vi "Write Nested Libraries.vi"(8 "error in (no error)":errorcluster, 10 "Nested Libraries":T1[](array[typedef]), 11 "TAF Proj Document Type:FrontPanelGUI in":refnum<class "FrontPanelGUI.lvclass">) -> (0 "error out":errorcluster, 3 "TAF Proj Document Type:FrontPanelGUI out":refnum<class "FrontPanelGUI.lvclass">)   [LabVIEW 2021]
uses:
  <vilib>/Wovalab/AntiDoc/Document Type/Add-ons/LabVIEW YAF Project/FrontPanelGUI/FrontPanelGUI.lvclass
  C:/Program Files (x86)/National Instruments/LabVIEW 2021/vi.lib/Wovalab/AntiDoc/Bloc/Bloc.lvclass
  C:/Program Files (x86)/National Instruments/LabVIEW 2021/vi.lib/Wovalab/AntiDoc/Document Type/Add-ons/LabVIEW YAF Project/FrontPanelGUI/FrontPanelGUI.lvclass
  <vilib>/Wovalab/AntiDoc/Document Type/Add-ons/LabVIEW YAF Project/FrontPanelGUI/Nested Lib Info--cluster.ctl
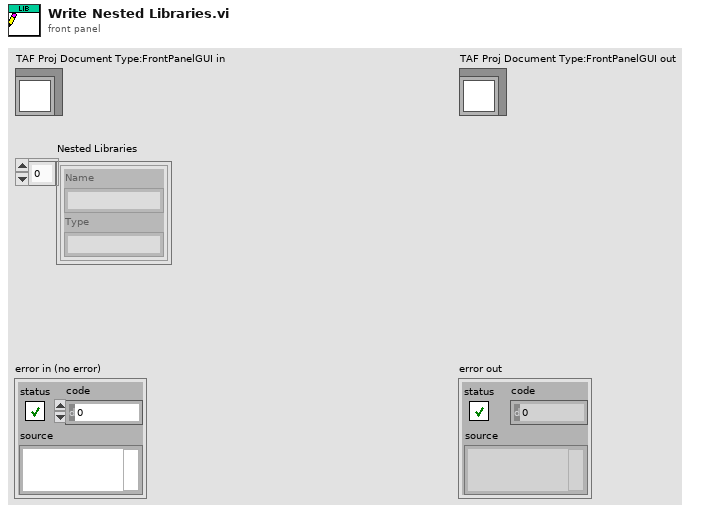
[diagram p1: front panel]
types:
  T1 = typedef "TAF Proj Document Type.lvlib/FrontPanelGUI.lvclass/Nested Lib Info--cluster.ctl" = cluster{"Name":string, "Type":string}
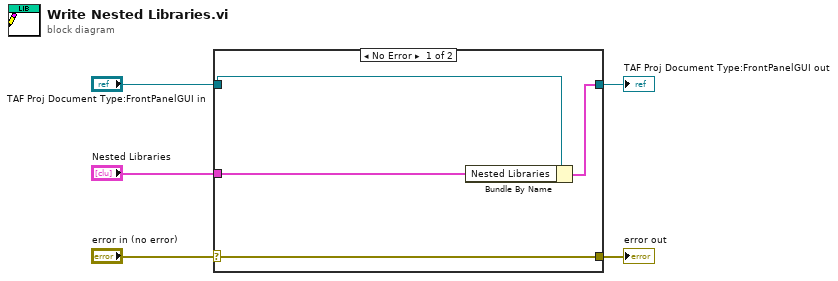
[diagram p0: block diagram]
diagram:
  n1 = case shown="No Error" "error in (no error)" {
    selector: "error in (no error)" -> [w9 w10]
    tunnel: [w9 w10] -> w4
    tunnel: [w7 w11] -> w2
    tunnel: "TAF Proj Document Type:FrontPanelGUI in" -> [w8 w11]
    tunnel: "Nested Libraries" -> [w6 _]
    frame No Error {
      n2 = Bundle By Name(cluster=w8, "Nested Libraries"=w6) -> (w7:cluster{})
    }
    frame Error {
    }
  }
  "error out" <- w4
  "TAF Proj Document Type:FrontPanelGUI out" <- w2
